vi "Read All Title Name.vi"(8 "error in (no error)":errorcluster, 11 "File String":string) -> (0 "error out":errorcluster, 3 "Title Name and Frame Num":cluster{"Name":string, "Num":i32}[](array[cluster]))   [LabVIEW 2018, in "Data Parser.lvclass"]
uses:
  Data Parser.lvclass
panel:
  out "frame num":i32
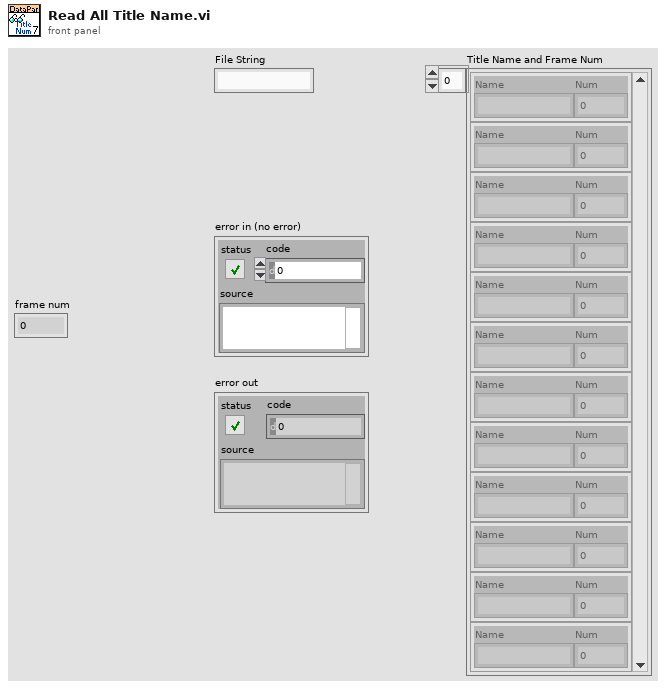
[diagram p1: front panel]
types:
  T1 = typedef "Data Parser.lvclass/frame data.ctl" = cluster{"Title":T2, "Basic Data":T3, "Sound":string, "<o> Data":T4, "<bp> Data":T5, "<c> Data":T6, "<w> Data":T7, "<i> Data Array":T8[], "<b> Data Array":T9[]}
  T2 = typedef "Data Parser.lvclass/frame title.ctl" = cluster{"Number":string, "Name":string}
  T3 = typedef "Data Parser.lvclass/frame basic data.ctl" = cluster{"Basic":cluster{"pic":string, "state":string, "wait":string, "next":string}, "Move":cluster{"dvx":string, "dvy":string, "dvz":string}, "Pic Center":cluster{"centerx":string, "centery":string}, "Skill":cluster{"hit_a":string, "hit_d":string, "hit_j":string, "hit_Fa":string, "hit_Ua":string, "hit_Da":string, "hit_Fj":string, "hit_Uj":string, "hit_Dj":string, "hit_ja":string}, "Mp":string}
  T4 = typedef "Data Parser.lvclass/frame o data.ctl" = cluster{"kind":string, "x":string, "y":string, "action":string, "dvx":string, "dvy":string, "dvz":string, "oid":string, "facing":string}
  T5 = typedef "Data Parser.lvclass/frame bp data.ctl" = cluster{"x":string, "y":string}
  T6 = typedef "Data Parser.lvclass/frame c data.ctl" = cluster{"kind":string, "x":string, "y":string, "injury":string, "cover":string, "vaction":string, "aaction":string, "taction":string, "hurtable":string, "decrease":string, "fronthurtact":string, "backhurtact":string, "dircontrol":string, "throwvx":string, "throwvy":string, "throwvz":string, "throwinjury":string}
  T7 = typedef "Data Parser.lvclass/frame w data.ctl" = cluster{"kind":string, "x":string, "y":string, "weaponact":string, "dvx":string, "dvy":string, "dvz":string, "attacking":string, "cover":string}
  T8 = typedef "Data Parser.lvclass/frame i data.ctl" = cluster{"kind":string, "x":string, "y":string, "w":string, "h":string, "dvx":string, "dvy":string, "dvz":string, "fall":string, "arest":string, "vrest":string, "bdefend":string, "injury":string, "zwidth":string, "effect":string, "catchingact":string, "caughtact":string}
  T9 = typedef "Data Parser.lvclass/frame b data.ctl" = cluster{"kind":string, "x":string, "y":string, "w":string, "h":string}
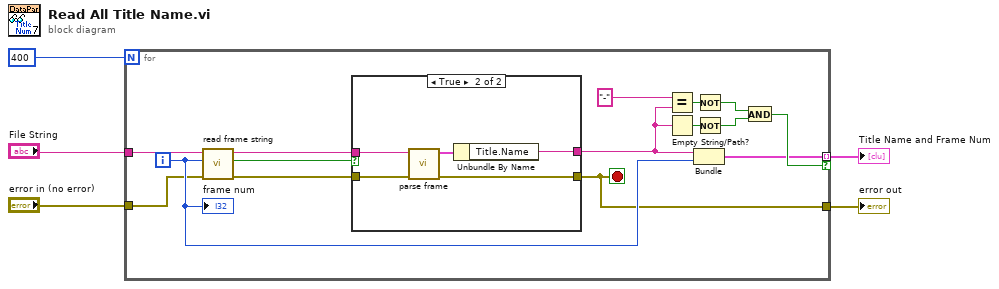
[diagram p0: block diagram]
diagram:
  n1 = for {
    N: 400 -> [_]
    tunnel: "File String" -> [w19]
    tunnel: [w8] -> w4 mode=indexing if=w11
    tunnel: "error in (no error)" -> [w7]
    tunnel: [w6] -> w1
    i -> [w9]
    stop <- w6 stop-if-true
    n2 = call "read frame string.vi"("error in"=w7, "frame number"=w9, "file string"=w19) -> ("error out"=w20:errorcluster, "found"=w18:bool, "<f> string"=w17:string)  [unwired: 5 in, 1 out]
    n3 = case shown="True" w18 {
      tunnel: w17 -> [_ w26]
      tunnel: w20 -> [w21 w25]
      tunnel: [w21 w22] -> w6
      tunnel: [_ w23] -> w10
      frame False {
      }
      frame True {
        n4 = call "parse frame.vi"("error in (no error)"=w25, "<f> string"=w26) -> ("error out"=w22:errorcluster, "frame data"=w24:T1)  [unwired: 8 in]
        n5 = Unbundle By Name(w24) -> ("Title.Name"=w23:string)
      }
    }
    n6 = Equal?(x="-", y=w10) -> (x = y?=w15:bool)
    n7 = Empty String/Path?(string/path=w10) -> (empty?=w14:bool)
    n8 = Bundle("Name"=w10, w9) -> (w8:cluster{"Name":string, i32})  [unwired: 1 in]
    n9 = Not(x=w15) -> (.not. x?=w13:bool)
    n10 = Not(x=w14) -> (.not. x?=w12:bool)
    n11 = And(x=w13, y=w12) -> (x .and. y?=w11:bool)
    "frame num" <- w9
  }
  "Title Name and Frame Num" <- w4
  "error out" <- w1
